vi "PicoScope3000aGetValues.vi"(5 "Segment Range":T1 {"toSegmentIndex" format="%.4p"; "fromSegmentIndex" format="%.4p"}, 7 "Buffer and Transfer Settings":T2={"startIndex"=0, "Samples"=1000, "Down Sample Ratio"=1, "Down-Sample Mode"=1} {"Down-Sample Mode" items=["RAW none"=2147483648, "None"=0, "Aggregate"=1, "Decimate"=2, "Average"=4]; "Down Sample Ratio" step=1; "Samples" format="%_6p"}, 8 "error in (no error)":errorcluster, 11 "handle in":i16) -> (0 "error out":errorcluster, 3 "handle out":i16, 4 "overflow":i16 format="%010b", 6 "noOfSamples":u64)   [LabVIEW 2010]
doc: "Calls ps5000aGetValuesOverlapped"
uses:
  ps3000a.dll
  shared/Buffer and Transfer Settings.ctl
  shared/Segment Range.ctl
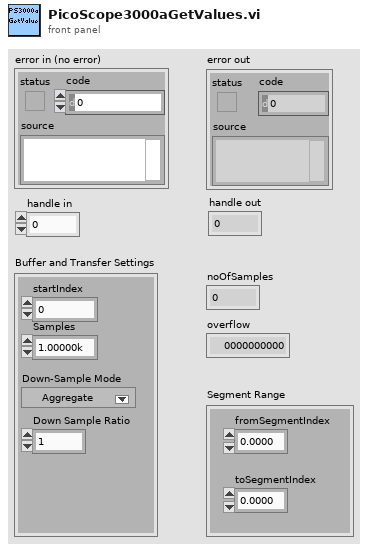
[diagram p1: front panel]
types:
  T1 = typedef "Segment Range.ctl" = cluster{"fromSegmentIndex":u64, "toSegmentIndex":u64}
  T2 = typedef "Buffer and Transfer Settings.ctl" = cluster{"startIndex":u64, "Samples":u64, "Down Sample Ratio":u64, "Down-Sample Mode":u32}
  T3 = cluster{"status":bool, "code":u32, "source":string}
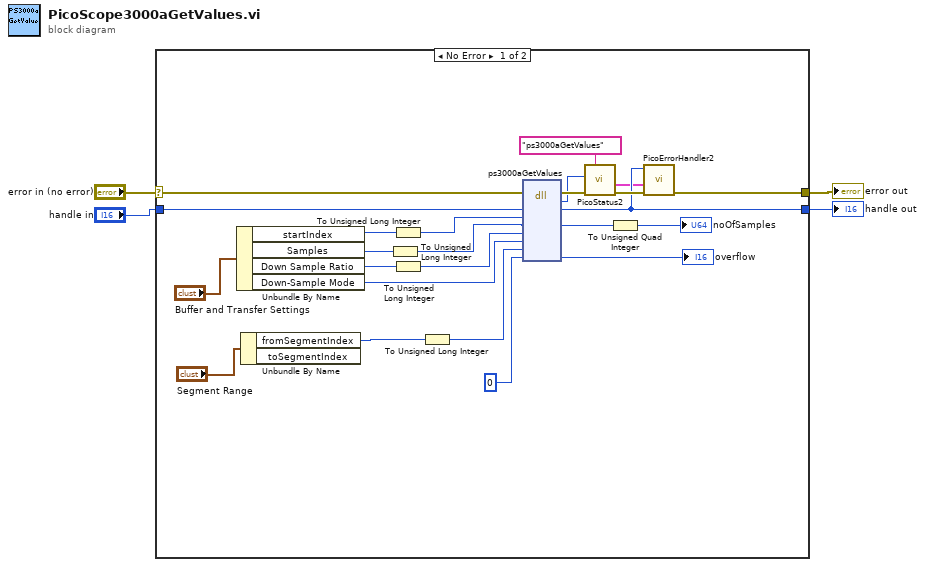
[diagram p0: block diagram]
diagram:
  n1 = case shown="No Error" "error in (no error)" {
    selector: "error in (no error)" -> [w23 w29]
    tunnel: "handle in" -> [w22 w30]
    tunnel: [w9 w30] -> w4
    tunnel: [w21 w29] -> w3
    frame No Error {
      n2 = Unbundle By Name("Buffer and Transfer Settings") -> ("startIndex"=w16:u64, "Samples"=w14:u64, "Down Sample Ratio"=w15:u64, "Down-Sample Mode"=w10:u32)
      n3 = Unbundle By Name("Segment Range") -> ("fromSegmentIndex"=w18:u64)  [unwired: 1 out]
      n4 = To Unsigned Long Integer(number=w14) -> (unsigned 32bit integer=w12:u32)
      n5 = To Unsigned Long Integer(number=w16) -> (unsigned 32bit integer=w13:u32)
      n6 = To Unsigned Long Integer(number=w15) -> (unsigned 32bit integer=w11:u32)
      n7 = To Unsigned Long Integer(number=w18) -> (unsigned 32bit integer=w17:u32)
      n8 = dll-call lib="ps3000a.dll" fn="ps3000aGetValues" ("ps3000.dll:_ps3000_open_unit@0")(error in=w23, "handle"=w22, "startIndex"=w13, "noOfSamples"=w12, "downSampleRatio"=w11, "downSampleRatioMode"=w10, "segmentIndex"=w17, "overflow"=i16 0) -> (error out=w27:errorcluster, "PICO_STATUS"=w5:u32, "handle"=w9:i16, "noOfSamples"=w8:u32, "overflow"=→"overflow":i16)  [unwired: 6 in, 1 out]
      n9 = call "PicoStatus2.vi"("PICO source"="ps3000aGetValues" ("source"), "Error in"=w27, "PICO STATUS"=w5) -> ("error out"=w28:errorcluster, "PICO_STATUS out"=w6:T3)  [unwired: 5 in]
      n10 = To Unsigned Quad Integer(1:w8) -> (0:→"noOfSamples":u64)
      n11 = call "PicoErrorHandler2.vi"("error in (no error)"=w28, "PICO_STATUS in"=w6, "handle In"=w9) -> ("error out"=w21:errorcluster)  [unwired: 8 in]
    }
    frame Error {
    }
  }
  "error out" <- w3
  "handle out" <- w4
